vi "Homogeneity_Score.vi"(8 "error in (no error)":errorcluster caption="entrée d'erreur (pas d'erreur)", 10 "labels_pred":string[][](array[string]), 11 "labels_true":string[][](array[string])) -> (0 "error out":errorcluster caption="sortie d'erreur", 3 "Score":string)   [LabVIEW 2020]
doc: "Homogeneity metric of a cluster labeling given a ground truth.\n\nA clustering result satisfies homogeneity if all of its clusters contain only data points which are members of a single class.\n\nThis metric is independent of the absolute values of the labels: a permutation of the class or cluster label values won’t change the score value in any way.\n\nThis metric is not symmetric: switching label_true with label_pred will return the completeness_score which will be different in general.\n\n\nParameters : \n\n- labels_true : int array, shape = [n_samples]\nground truth class labels to be used as a reference\n\n- labels_pred : array-like of shape (n_samples,)\ncluster labels to evaluate\n\nReturns : \n\n- homogeneity : float\nscore between 0.0 and 1.0. 1.0 stands for perfectly homogeneous labeling"
uses:
  Homogeneity_Score.lvclass
panel:
  out "Homogeneity_Score.lvclass":refnum<class "Homogeneity_Score.lvclass">
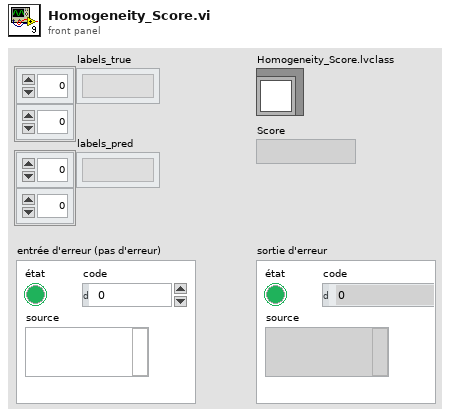
[diagram p1: front panel]
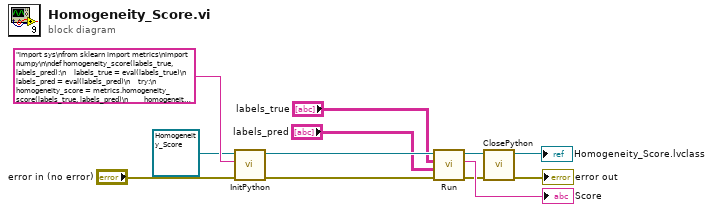
[diagram p0: block diagram]
diagram:
  n1 = call-dynamic "InitPython.vi"("error in (no error)"="error in (no error)", "Python Instruction"="import sys\nfrom sklearn import metrics\nimport numpy\n\ndef homogeneity_score(labels_true, labels_pred):\n    labels_true = eval(labels_true)\n    labels_pred = eval(labels_pred)\n    try:\n        homogeneity_score = metrics.homogeneity_score(labels_true, labels_pred)\n        homogeneity_score = homogeneity_score.tolist()\n        return str(homogeneity_score)\n    except:\n        erreur = sys.exc_info()\n        typerr = u\"%s\" % (erreur[0])\n        typerr = typerr[typerr.find(\"'\")+1:typerr.rfind(\"'\")]\n        msgerr = u\"%s\" % (erreur[1])\n        message = str('/!\\\\ {0} : {1}'. format(typerr,msgerr))\n        return message", "Scikit-learn en entrée"=refnum<class "Homogeneity_Score.lvclass"> refnum ("Homogeneity_Score.lvclass")) -> ("error out"=w7:errorcluster, "Scikit-learn en sortie"=w8:refnum<class "Homogeneity_Score.lvclass">)  [unwired: 7 in]
  n2 = call-dynamic "Run.vi"("error in (no error)"=w7, "labels_pred"="labels_pred", "labels_true"="labels_true", "Homogeneity_Score.lvclass"=w8) -> ("error out"=w4:errorcluster, "String Data"=→"Score":string, "Homogeneity_Score.lvclass"=w6:refnum<class "Homogeneity_Score.lvclass">)  [unwired: 5 in]
  n3 = call-dynamic "ClosePython.vi"("error in (no error)"=w4, "Scikit-learn en entrée"=w6) -> ("error out"=→"error out":errorcluster, "Scikit-learn en sortie"=→"Homogeneity_Score.lvclass":refnum<class "Homogeneity_Score.lvclass">)  [unwired: 8 in]
